vi "Measurement UI.vi"() -> ()   [LabVIEW 2023, in "FPT Intermodulation UI.lvlib"]
uses:
  FPT Intermodulation UI.lvlib
panel:
  in  "Measurement Graph":T1(tab)
  out "Graph Combined":T2(graph)
  out "Graph DUT Gain":T2(graph)
  out "Graph Intermodulation":T2(graph)
  out "Graph TOI":T2(graph)
  out "Graph Fundamental":T2(graph)
  out "TS_Intermodulation Slope (dBm)":dbl[][](array[numeric])
  out "TS_Fundamental Slope (dBm)":dbl[][](array[numeric])
  out "Final Target Pout (dBm)":dbl
  out "All Data":dbl[][](array[numeric])
  out "TS_DUT Gain (dBm)":dbl[][](array[numeric])
  out "TS_TOI (dBm)":dbl[][](array[numeric])
  out "TS_IMD (dBm)":dbl[][](array[numeric])
  out "TS_Fundamental (dBm)":dbl[][](array[numeric])
  out "Typical OIP3 (dBm)":dbl
  out "x-axis label":string
  in  "Power sequencing file path":string
  in  "RFSG name":string="5842_0"
  in  "RFSG attenuation mode":T3(ring)=enum."Constant Attenuation"
  in  "RFSG s2p file path":string
  in  "RFmx name":string="5842_0"
  in  "RFmx attenuation mode":T3(ring)=enum."Constant Attenuation"
  in  "RFmx s2p file path":string
  out "All Graph Reference":refnum<vi>[](array[refnum])
  out "All Plots Data":T4(array[cluster])
  in  "IM_Sweep Mode":enum32{"Power", "Frequency", "Tone Spacing"}(ring) caption="Sweep Mode"
  out "MeasTable_Fix":string[][](table)
  out "MeasTable":string[][](table)
  in  "Tab Control":T5(tab)
  in  "Power sequencing file path_update":path caption="Power Sequencing File Path"
  in  "RFSG name_update":refnum<k15> caption="RFSG Name"
  in  "RFSG attenuation mode_tab":T3(tab)=enum."s2p File" caption="RFSG Attenuation Mode"
  in  "RFSG external attenuation (dB)":dbl caption="External Attenuation" format="%#.3pdB"
  in  "RFSG s2p file path_update":path caption="S2P File Path"
  in  "RFSG s-parameters orientation":enum32{"Port1 Towards DUT", "Port2 Towards DUT"}(ring) caption="Orientation"
  in  "RFmx name_update":refnum<k15> caption="RFmx Name"
  in  "RFmx attenuation mode_tab":T3(tab) caption="RFmx Attenuation Mode"
  in  "RFmx external attenuation (dB)":dbl caption="External Attenuation" format="%#.3pdB"
  in  "RFmx s2p file path_update":path caption="S2P File Path"
  in  "RFmx s-parameters orientation":enum32{"Port1 Towards DUT", "Port2 Towards DUT"}(ring) caption="Orientation"
  in  "RFSG port":string(combo)="port1" caption="RFSG Port"
  in  "RFmx port":string(combo)="port2" caption="RFmx Port"
  in  "RFmx Reference Level (dBm)":dbl=10.0 caption="Reference Level" format="%#.3fdBm"
  in  "RFSG Generation IQ Rate (S/s)":dbl=1250000000.0 caption="Generation IQ Rate" format="%#.3pS/s"
  in  "Start Pin Per Tone (dBm)":dbl=-20.0 caption="Start Pin Per Tone" format="%#.3fdBm"
  in  "Start Center Frequency (Hz)":dbl=8000000000.0 caption="Start Center Frequency" format="%#.3pHz"
  in  "Start Tone Spacing (Hz)":dbl=1000000.0 caption="Start Tone Spacing" format="%#.3pHz"
  in  "Sweep Delay (ms)":u32 format="%#.3pms"
  in  "Sweep Mode_tab":enum32{"Power", "Frequency", "Tone Spacing"}(tab)=enum."Tone Spacing" caption="Sweep Mode"
  in  "Power Sweep End":dbl format="%#.fdBm"
  in  "Power Sweep Step":dbl=1.0 format="%#.fdB"
  in  "Target Pout Per Tone (dBm)":dbl caption="Target Pout Per Tone" format="%#.3fdBm"
  in  "Frequency Sweep End":dbl=12000000000.0 format="%#.pHz"
  in  "Frequency Sweep Step":dbl=100000000.0 format="%#.pHz"
  in  "Tone Spacing Sweep End":dbl=10000000.0 format="%#.pHz"
  in  "Tone Spacing Sweep Step":dbl=1000000.0 format="%#.pHz"
  in  "Mode of operation":T6(ring) caption="Configuration"
  out "Status":string
  # "Intermodulation"
  # "Sweep Options"
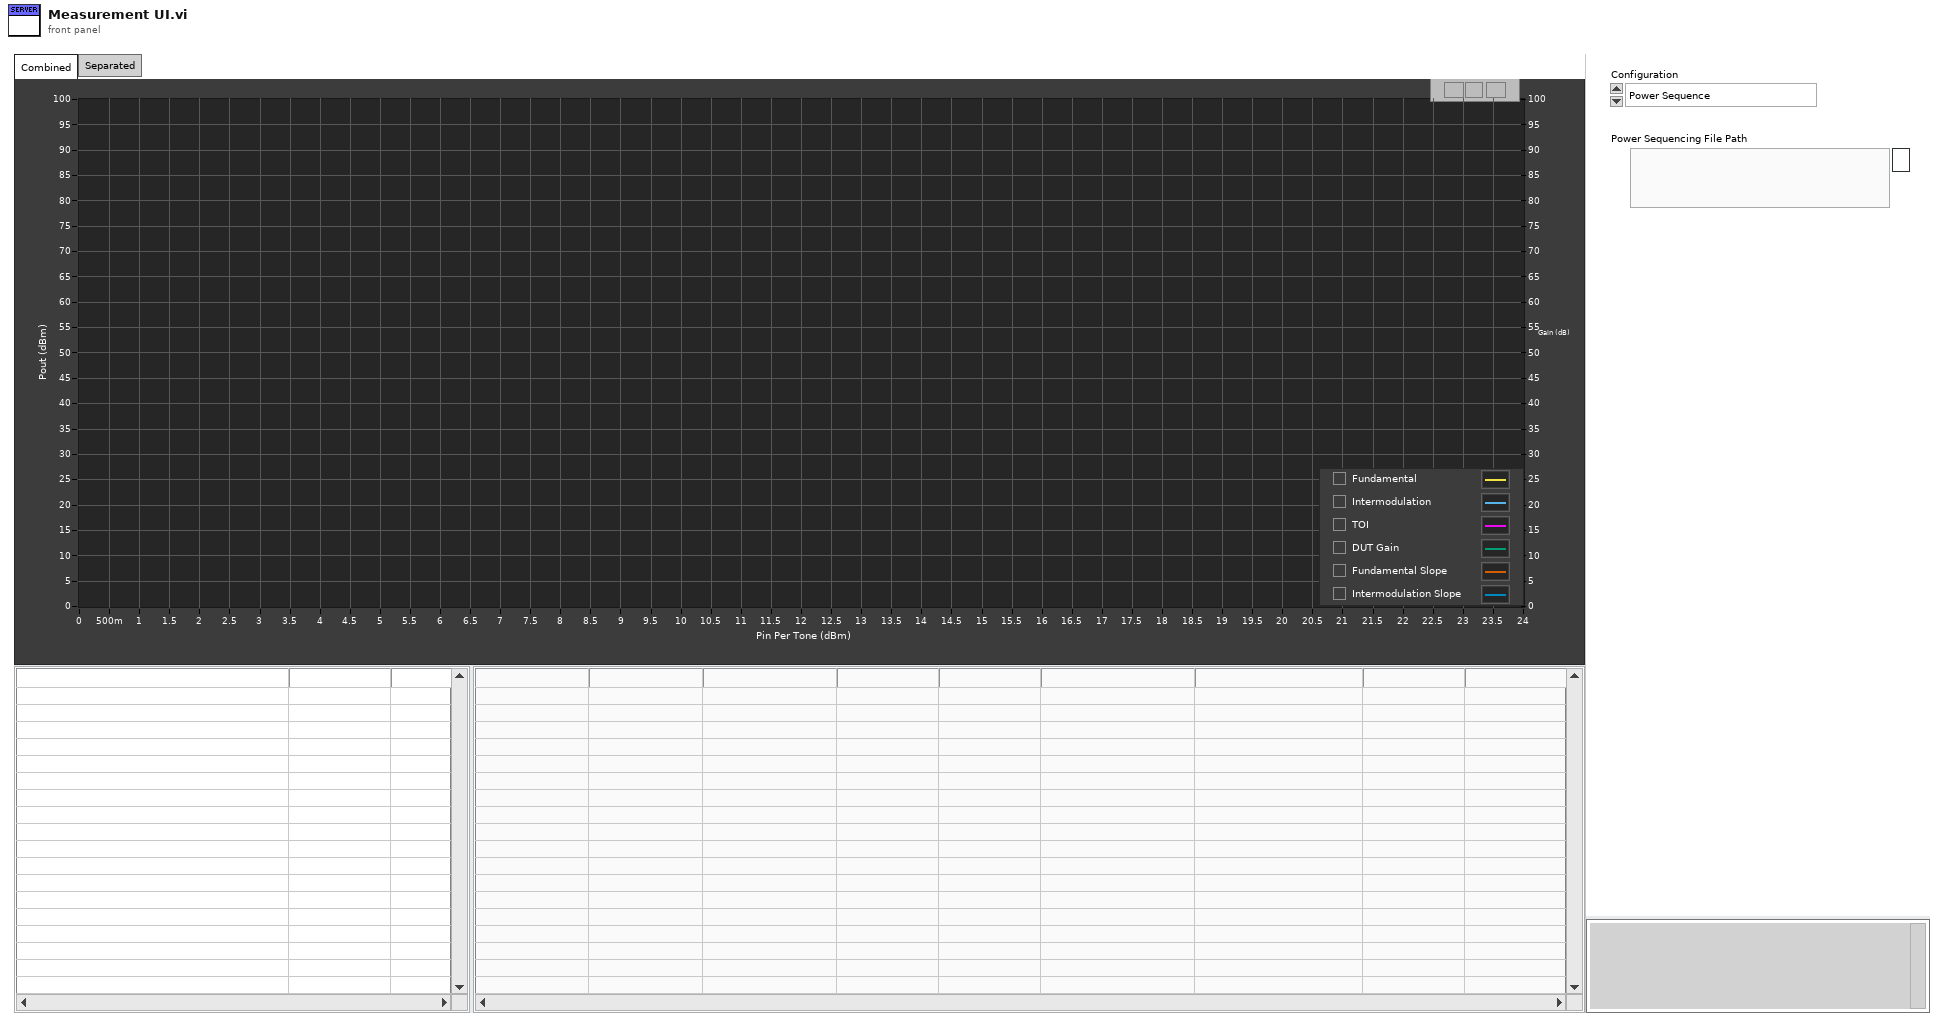
[diagram p1: front panel]
types:
  T1 = enum32{"Combined", "Separated", "Hidden Controls"}
  T2 = cluster{"Load currents":dbl[], "Efficiency":dbl[]}[]
  T3 = enum32{"<None>", "Constant Attenuation", "s2p File"}
  T4 = cluster{"X-axis values":dbl[], "Y-axis values":dbl[]}[]
  T5 = enum32{"Power Sequence", "Correction", "Measurement 1"}
  T6 = enum32{"Power Sequence", "HW + Correction", "Measurement 1"}
  T7 = enum8{"Enabled", "Disabled", "Disabled and Grayed Out"}
  T8 = cluster{"Shift":bool, "Ctrl":bool, "Alt":bool, "Cmd":bool, "Opt":bool}
  T9 = cluster{"TS_Fundamental Slope (dBm)":dbl[], "TS_Fundamental Slope (dBm)":dbl[]}
  T10 = cluster{"TS_Fundamental Slope (dBm)":dbl[], "TS_Intermodulation Slope (dBm)":dbl[]}
  T11 = cluster{"TS_Fundamental Slope (dBm)":dbl[], "TS_Intermodulation Slope (dBm)":dbl[]}[]
  T12 = cluster{"TS_Fundamental (dBm)":dbl[], "TS_Fundamental (dBm)":dbl[]}
  T13 = cluster{"TS_Fundamental (dBm)":dbl[], "TS_IMD (dBm)":dbl[]}
  T14 = cluster{"TS_Fundamental (dBm)":dbl[], "TS_TOI (dBm)":dbl[]}
  T15 = cluster{"TS_Fundamental (dBm)":dbl[], "TS_DUT Gain (dBm)":dbl[]}
  T16 = cluster{"X-axis values":dbl[], "Y-axis values":dbl[]}
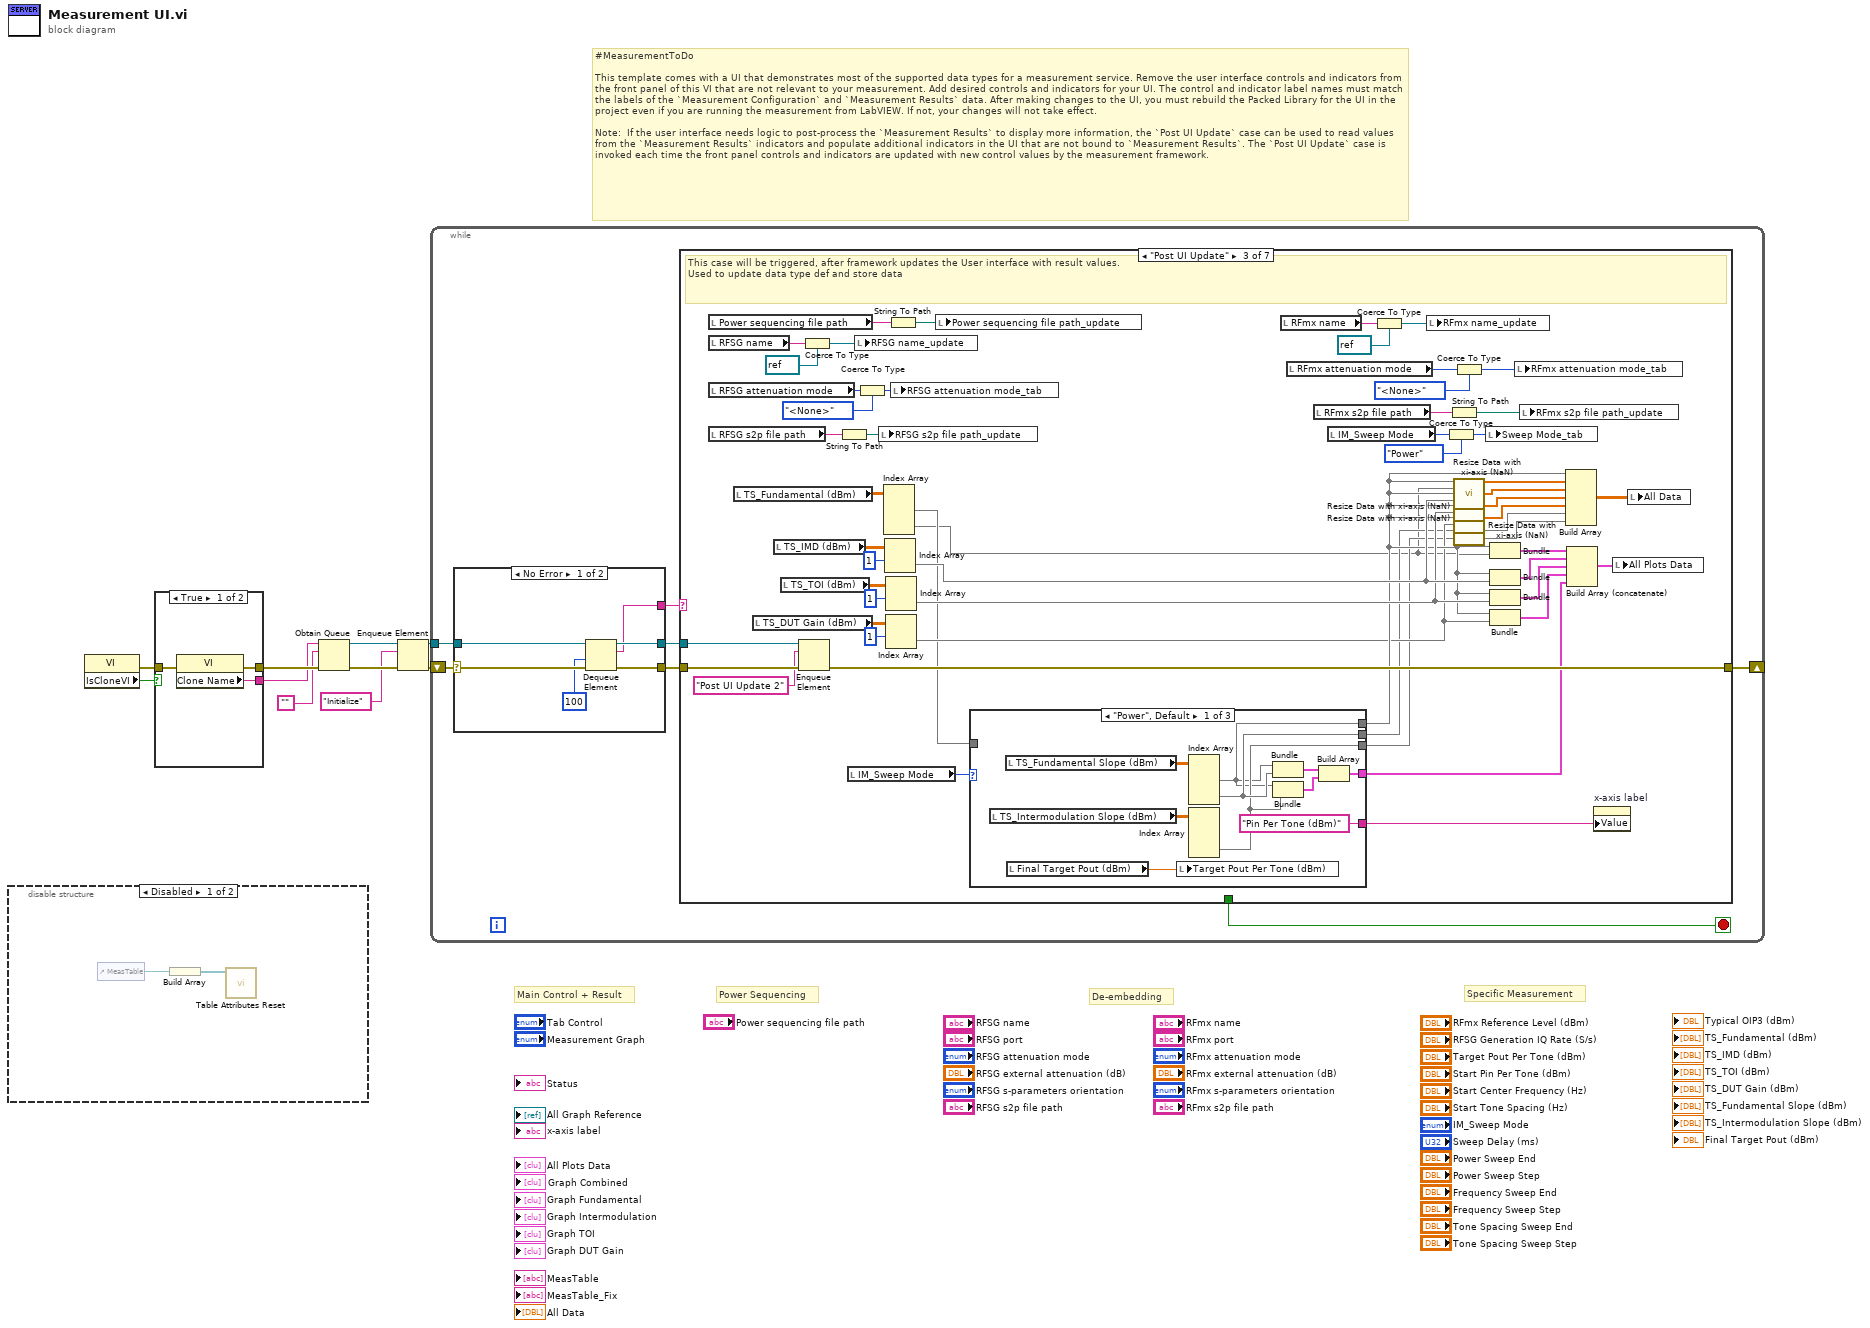
[diagram p0: block diagram]
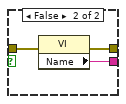
[diagram p3: hidden frame]
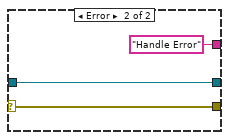
[diagram p4: hidden frame]
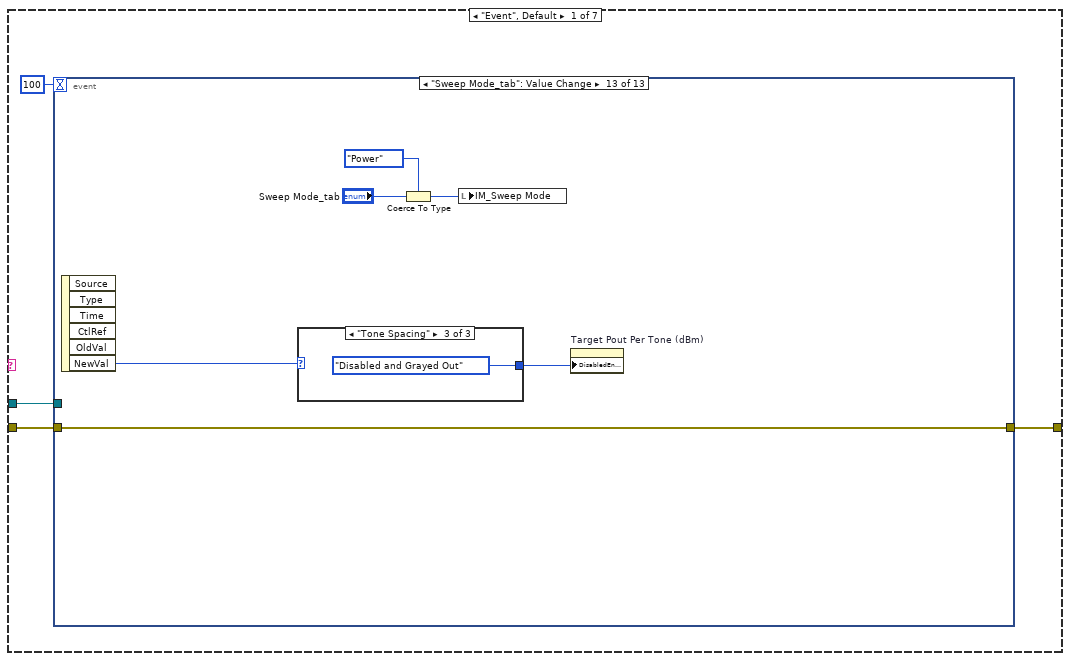
[diagram p5: hidden frame]
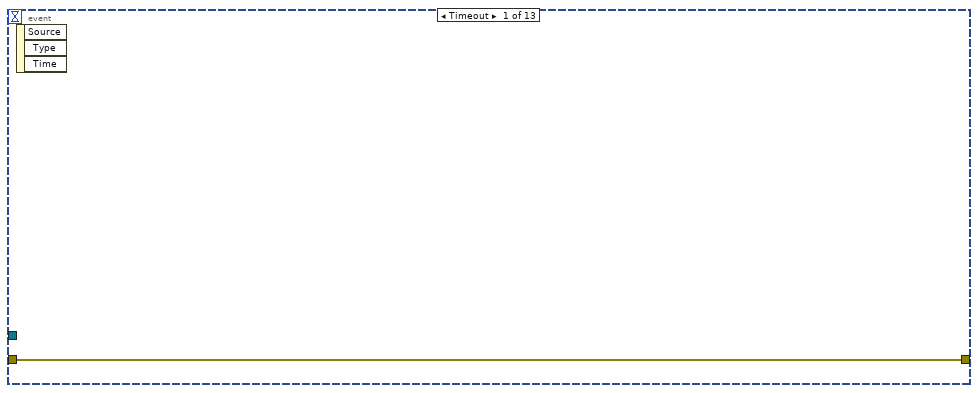
[diagram p6: hidden frame]
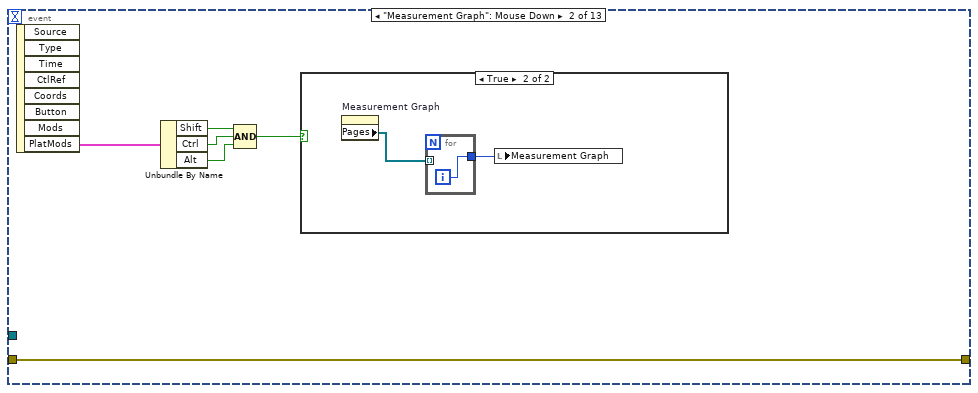
[diagram p7: hidden frame]
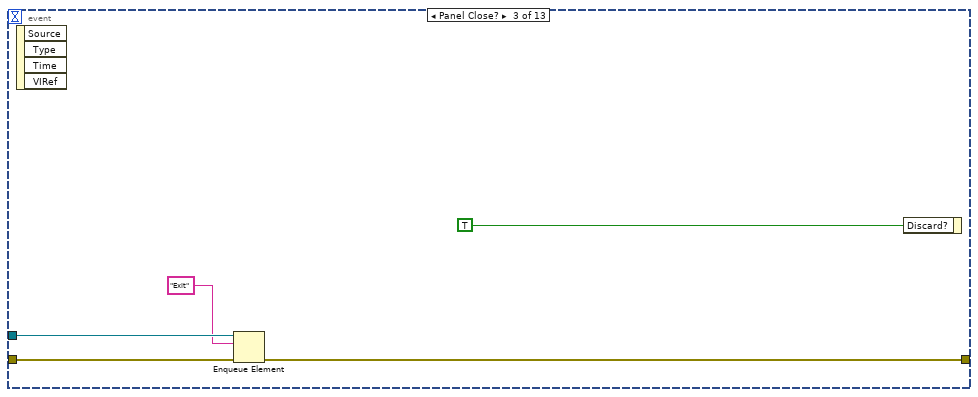
[diagram p9: hidden frame]
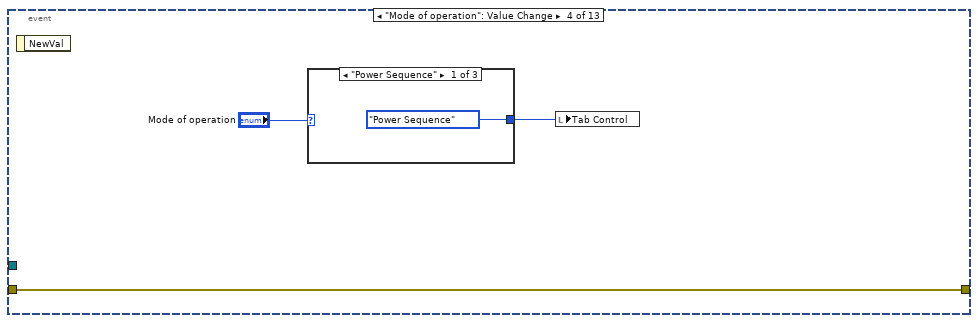
[diagram p10: hidden frame]
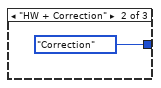
[diagram p11: hidden frame]
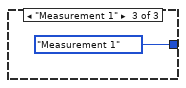
[diagram p12: hidden frame]
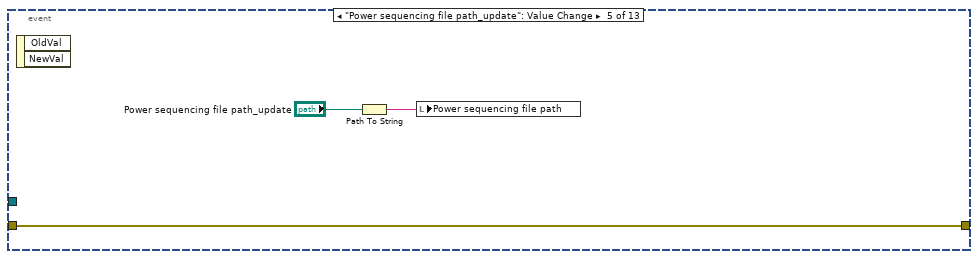
[diagram p13: hidden frame]
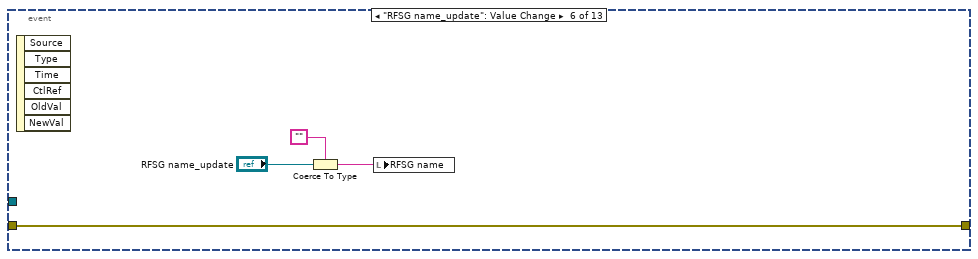
[diagram p14: hidden frame]
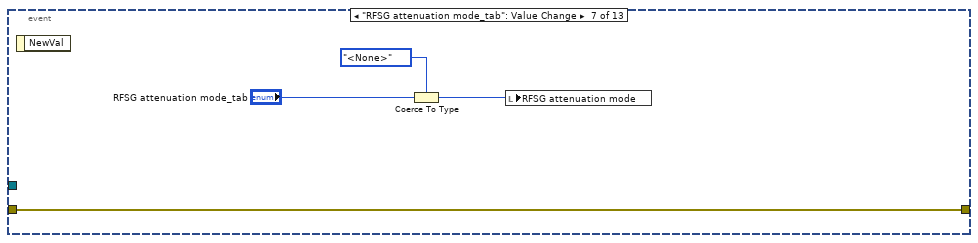
[diagram p15: hidden frame]
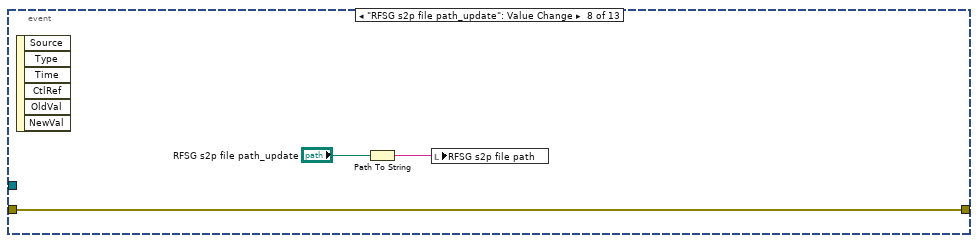
[diagram p16: hidden frame]
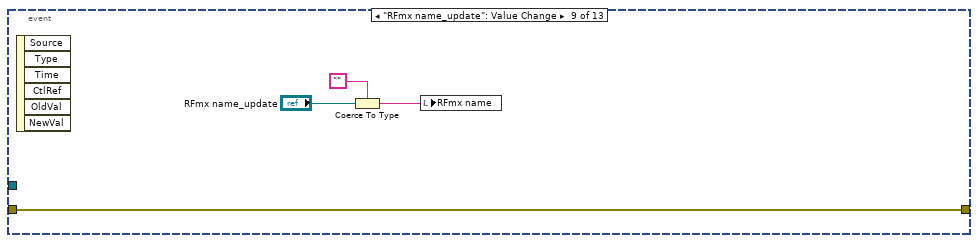
[diagram p17: hidden frame]
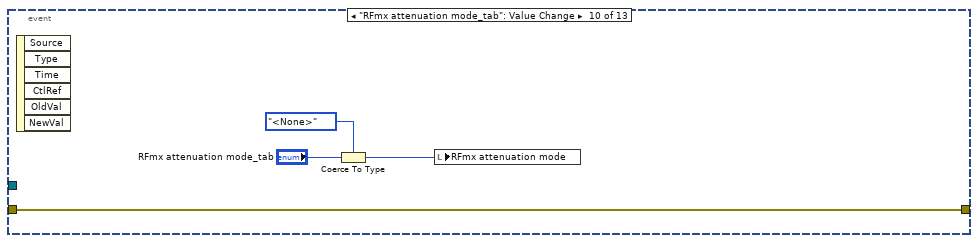
[diagram p18: hidden frame]
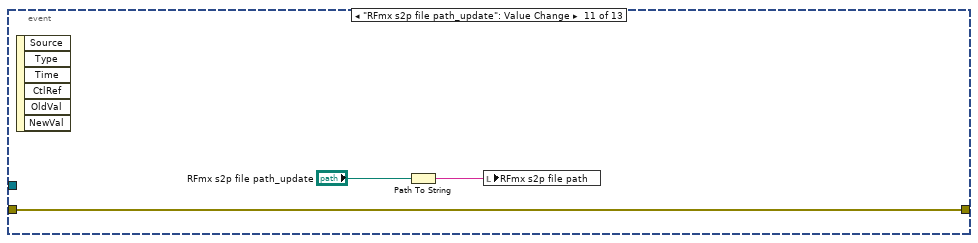
[diagram p19: hidden frame]
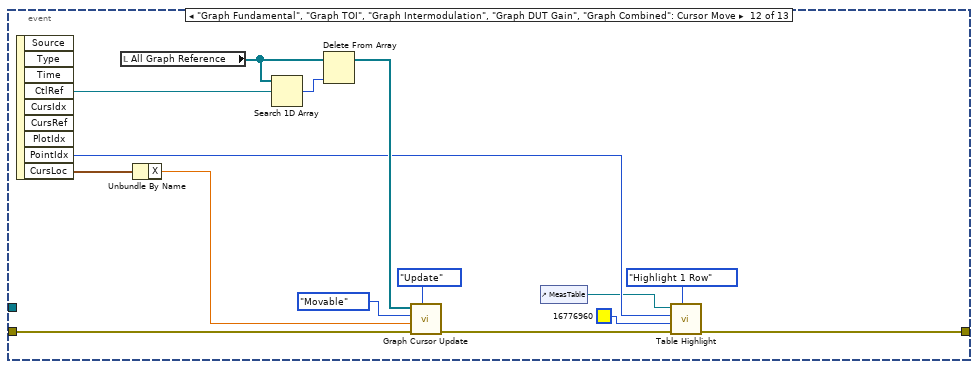
[diagram p20: hidden frame]
diagram:
  # "Specific Measurement"
  # "De-embedding"
  # "Power Sequencing"
  # "Main Control + Result"
  # "#MeasurementToDo  \n\nThis template comes with a UI that demonstrates most of the supported data types for a measurement service. Remove the user interface controls and indicators from the front panel of this VI that are not relevant to your measurement. Add desired controls and indicators for your UI. The control and indicator label names must match the labels of the `Measurement Configuration` and `Measurement Results` data. After making changes to the UI, you must rebuild the Packed Library for the UI in the project even if you are running the measurement from LabVIEW. If not, your changes will not take effect.\n\nNote:  If the user interface needs logic to post-process the `Measurement Results` to display more information, the `Post UI Update` case can be used to read values from the `Measurement Results` indicators and populate additional indicators in the UI that are not bound to `Measurement Results`. The `Post UI Update` case is invoked each time the front panel controls and indicators are updated with new control values by the measurement framework."
  n1 = disable-structure shown="Disabled" {
    frame Disabled {
      n2 = control-ref of="MeasTable"() -> (w12:refnum<vi>)
      n3 = Build Array(w12) -> (w11:refnum<vi>[])
      n4 = call "Table Attributes Reset.vi"("Table Refs"=w11) -> ()  [unwired: 11 in]
    }
    frame Enabled {
    }
  }
  n5 = property class="VI"() -> (error out=w1:errorcluster, "IsCloneVI"=w2:bool)  [unwired: 2 in, 1 out]
  n6 = case shown="True" w2 {
    tunnel: [w15 w18] -> w10
    tunnel: [w14 w17] -> w9
    tunnel: w1 -> [w13 w16]
    frame True {
      n7 = property class="VI"(error in=w13) -> (error out=w15:errorcluster, "Clone Name"=w14:string)  [unwired: 1 in, 1 out]
    }
    frame False {
      n8 = property class="VI"(error in=w16) -> (error out=w18:errorcluster, "Name"=w17:string)  [unwired: 1 in, 1 out]
    }
  }
  n9 = Obtain Queue(name (unnamed)=w9, element data type="", error in (no error)=w10) -> (queue out=w6:refnum<queue>, error out=w8:errorcluster)  [unwired: 2 in, 1 out]
  n10 = Enqueue Element(queue=w6, element="Initialize", error in (no error)=w8) -> (queue out=w5:refnum<queue>, error out=w7:errorcluster)  [unwired: 1 in, 1 out]
  n11 = while {
    shift-right: [w20] -> _
    shift-left: w7 -> [w25]
    tunnel: w5 -> [w23]
    stop <- w19 stop-if-true
    n12 = case shown="No Error" w25 {
      selector: w25 -> [w31 w34]
      tunnel: [w30 w34] -> w24
      tunnel: w23 -> [w29 w33]
      tunnel: [w28 w33] -> w22
      tunnel: [w27 "Handle Error"] -> w21
      frame No Error {
        n13 = Dequeue Element(queue=w29, timeout in ms (-1)=100, error in (no error)=w31) -> (queue out=w28:refnum<queue>, element=w27:string, error out=w30:errorcluster)  [unwired: 1 out]
      }
      frame Error {
      }
    }
    n14 = case shown="\"Post UI Update\"" w21 {
      tunnel: w24 -> [w37 w120 w172 w213 w237 w251 w252]
      tunnel: w22 -> [w35 _ w171 w212 _ w249 _]
      tunnel: [w38 w120 w172 w202 w237 w246 w252] -> w20
      tunnel: [_ _ _ _ _ TRUE _] -> w19
      frame "Event", Default {
        n15 = event shown="[12] \"Sweep Mode_tab\": Value Change" {
          selector: _ -> [_ _ _ _ _ _ _ _ _ _ _ _ _]
          dyn-events: _ -> [_ _ _ _ _ _ _ _ _ _ _ _ _]
          timeout: 100 -> [_ _ _ _ _ _ _ _ _ _ _ _ _]
          tunnel: [w39 w45 w51 w55 w60 w63 w69 w71 w74 w80 w82 w89 w105] -> w38
          tunnel: w37 -> [w39 w45 w52 w55 w60 w63 w69 w71 w74 w80 w82 w99 w105]
          tunnel: w35 -> [_ _ w50 _ _ _ _ _ _ _ _ _ _]
          event Timeout {
            n16 = event-data() -> ()  [unwired: 1 in, 3 out]
          }
          event "Measurement Graph": Mouse Down {
            n17 = event-data() -> ("PlatMods"=w44:T8)  [unwired: 1 in, 7 out]
            n18 = Unbundle By Name(w44) -> ("Shift"=w43:bool, "Ctrl"=w42:bool, "Alt"=w41:bool)
            n19 = Compound Arithmetic op=AND(w43, w42, w41) -> (w40:bool)
            n20 = case shown="True" w40 {
              frame False {
              }
              frame True {
                n21 = property on="Measurement Graph" class="TabCtl (strict)"() -> ("Pages"=w47:refnum<vi>[])  [unwired: 2 in, 2 out]
                n22 = for {
                  tunnel: w47 -> [_] mode=indexing
                  tunnel: [w48] -> w46
                  i -> [w48]
                }
                n23 = local write "Measurement Graph"(w46) -> ()
              }
            }
          }
          event Panel Close? {
            n24 = event-data() -> ()  [unwired: 1 in, 4 out]
            n25 = Enqueue Element(queue=w50, element="Exit", error in (no error)=w52) -> (error out=w51:errorcluster)  [unwired: 1 in, 2 out]
            n26 = event-data("Discard?"=TRUE) -> ()  [unwired: 1 in, 1 out]
          }
          event "Mode of operation": Value Change {
            n27 = event-data() -> ()  [unwired: 1 in, 1 out]
            n28 = case shown="\"Power Sequence\"" "Mode of operation" {
              tunnel: [T5."Power Sequence" ("Tab Control") T5."Correction" ("Tab Control") T5."Measurement 1" ("Tab Control")] -> w54
              frame "Power Sequence" {
              }
              frame "HW + Correction" {
              }
              frame "Measurement 1" {
              }
            }
            n29 = local write "Tab Control"(w54) -> ()
          }
          event "Power sequencing file path_update": Value Change {
            n30 = event-data() -> ()  [unwired: 1 in, 2 out]
            n31 = Path To String(path="Power sequencing file path_update") -> (string=w61:string)
            n32 = local write "Power sequencing file path"(w61) -> ()
          }
          event "RFSG name_update": Value Change {
            n33 = event-data() -> ()  [unwired: 1 in, 6 out]
            n34 = Coerce To Type(0:"RFSG name_update", 1:"") -> (2:w64:string)
            n35 = local write "RFSG name"(w64) -> ()
          }
          event "RFSG attenuation mode_tab": Value Change {
            n36 = event-data() -> ()  [unwired: 1 in, 1 out]
            n37 = Coerce To Type(0:"RFSG attenuation mode_tab", 1:T3."<None>" ("RFSG attenuation mode")) -> (2:w68:T3)
            n38 = local write "RFSG attenuation mode"(w68) -> ()
          }
          event "RFSG s2p file path_update": Value Change {
            n39 = event-data() -> ()  [unwired: 1 in, 6 out]
            n40 = Path To String(path="RFSG s2p file path_update") -> (string=w72:string)
            n41 = local write "RFSG s2p file path"(w72) -> ()
          }
          event "RFmx name_update": Value Change {
            n42 = event-data() -> ()  [unwired: 1 in, 6 out]
            n43 = Coerce To Type(0:"RFmx name_update", 1:"") -> (2:w76:string)
            n44 = local write "RFmx name"(w76) -> ()
          }
          event "RFmx attenuation mode_tab": Value Change {
            n45 = event-data() -> ()  [unwired: 1 in, 6 out]
            n46 = Coerce To Type(0:"RFmx attenuation mode_tab", 1:T3."<None>" ("RFmx attenuation mode")) -> (2:w79:T3)
            n47 = local write "RFmx attenuation mode"(w79) -> ()
          }
          event "RFmx s2p file path_update": Value Change {
            n48 = event-data() -> ()  [unwired: 1 in, 6 out]
            n49 = Path To String(path="RFmx s2p file path_update") -> (string=w83:string)
            n50 = local write "RFmx s2p file path"(w83) -> ()
          }
          event "Graph Fundamental", "Graph TOI", "Graph Intermodulation", "Graph DUT Gain", "Graph Combined": Cursor Move {
            n51 = event-data() -> ("CtlRef"=w97:refnum<vi>, "PointIdx"=w87:i32, "CursLoc"=w98:cluster{"X":dbl, "Y":dbl})  [unwired: 1 in, 6 out]
            n52 = local read "All Graph Reference"() -> (w96:refnum<vi>[])
            n53 = Unbundle By Name(w98) -> ("X"=w92:dbl)
            n54 = Search 1D Array(1D array=w96, element=w97) -> (index of element=w95:i32)  [unwired: 1 in]
            n55 = Delete From Array(array=w96, index=w95) -> (array with subset deleted=w94:refnum<vi>[])  [unwired: 1 in, 1 out]
            n56 = call "Graph Cursor Update.vi"("Action"=enum16{"Reset", "Update"}."Update", "error in"=w99, "New X position"=w92, "Cursor Type"=enum16{"Movable", "Fixed", "All"}."Movable", "Graph Refs in"=w94) -> ("error out"=w90:errorcluster)  [unwired: 5 in, 1 out]
            n57 = control-ref of="MeasTable"() -> (w86:refnum<vi>)
            n58 = call "Table Highlight.vi"("Action"=enum16{"Reset", "Highlight 1 Row"}."Highlight 1 Row", "error in"=w90, "Color Box"=u32 16776960, "Row"=w87, "Table Ref in"=w86) -> ("error out"=w89:errorcluster)  [unwired: 5 in, 1 out]
          }
          event "Sweep Mode_tab": Value Change {
            n59 = event-data() -> ("NewVal"=w100:enum32{"Power", "Frequency", "Tone Spacing"})  [unwired: 1 in, 5 out]
            n60 = case shown="\"Tone Spacing\"" w100 {
              tunnel: [T7."Disabled and Grayed Out" ("Disabled") T7."Enabled" ("Disabled") T7."Disabled and Grayed Out" ("Disabled")] -> w101
              frame "Frequency" {
              }
              frame "Power" {
              }
              frame "Tone Spacing" {
              }
            }
            n61 = Coerce To Type(0:"Sweep Mode_tab", 1:enum32{"Power", "Frequency", "Tone Spacing"}."Power" ("IM_Sweep Mode")) -> (2:w102:enum32{"Power", "Frequency", "Tone Spacing"})
            n62 = local write "IM_Sweep Mode"(w102) -> ()
            n63 = property on="Target Pout Per Tone (dBm)" class="DigNum (strict)"("DisabledEnum"=w101) -> ()  [unwired: 2 in, 2 out]
          }
        }
      }
      frame "Initialize" {
        w115 = 0
        n64 = local write "Tab Control"(w115) -> ()
        n65 = local write "Mode of operation"(w115) -> ()
        n66 = control-ref of="Graph Combined"() -> (w114:refnum<vi>)
        n67 = control-ref of="Graph Fundamental"() -> (w119:refnum<vi>)
        n68 = control-ref of="Graph Intermodulation"() -> (w117:refnum<vi>)
        n69 = control-ref of="Graph TOI"() -> (w116:refnum<vi>)
        n70 = control-ref of="Graph DUT Gain"() -> (w118:refnum<vi>)
        n71 = Build Array(w114, w119, w117, w116, w118) -> (w113:refnum<vi>[])
        n72 = property on="All Graph Reference" class="Arr (strict)"("Value"=w113) -> ()  [unwired: 2 in, 2 out]
        n73 = call "Graph Set Cursor Mode.vi"("Cursor Mode"=enum32{"Free-Drag", "Single-Plot", "Multi-Plot"}."Multi-Plot", "Graph Refs in"=w113) -> ("Graph Refs out"=w111:refnum<vi>[])  [unwired: 8 in, 1 out]
        n74 = call "Graph Cursor Update.vi"("Action"=enum16{"Reset", "Update"}."Reset", "Cursor Type"=enum16{"Movable", "Fixed", "All"}."All", "Graph Refs in"=w111) -> ()  [unwired: 7 in, 2 out]
      }
      frame "Post UI Update" {
        # "This case will be triggered, after framework updates the User interface with result values.\nUsed to update data type def and store data"
        n75 = local read "Power sequencing file path"() -> (w168:string)
        n76 = local read "RFSG name"() -> (w166:string)
        n77 = local read "RFSG attenuation mode"() -> (w167:T3)
        n78 = local read "RFSG s2p file path"() -> (w162:string)
        n79 = local read "TS_Fundamental (dBm)"() -> (w122:dbl[][])
        n80 = local read "TS_DUT Gain (dBm)"() -> (w149:dbl[][])
        n81 = local read "TS_IMD (dBm)"() -> (w151:dbl[][])
        n82 = local read "TS_TOI (dBm)"() -> (w150:dbl[][])
        n83 = Enqueue Element(queue=w171, element="Post UI Update 2") -> ()  [unwired: 2 in, 3 out]
        n84 = Coerce To Type(0:w166, 1:refnum<k15> refnum ("RFSG name_update")) -> (2:w164:refnum<k15>)
        n85 = String To Path(string=w162) -> (path=w163:path)
        n86 = local read "IM_Sweep Mode"() -> (w123:enum32{"Power", "Frequency", "Tone Spacing"})
        n87 = local write "RFSG name_update"(w164) -> ()
        n88 = Coerce To Type(0:w167, 1:T3."<None>" ("RFSG attenuation mode_tab")) -> (2:w155:T3)
        n89 = local write "RFSG s2p file path_update"(w163) -> ()
        n90 = Index Array(array=w122) -> (element #1=w130:dbl[], element #2=w121:dbl[])  [unwired: 4 in]
        n91 = Index Array(array=w151, index (row)=1) -> (element=w138:dbl[])  [unwired: 1 in]
        n92 = Index Array(array=w150, index (row)=1) -> (element=w136:dbl[])  [unwired: 1 in]
        n93 = Index Array(array=w149, index (row)=1) -> (element=w133:dbl[])  [unwired: 1 in]
        n94 = String To Path(string=w168) -> (path=w169:path)
        n95 = local write "RFSG attenuation mode_tab"(w155) -> ()
        n96 = local write "Power sequencing file path_update"(w169) -> ()
        n97 = case shown="\"Power\", Default" w123 {
          tunnel: [w180 _ _] -> w132
          tunnel: [w177 _ _] -> w141
          tunnel: w130 -> [_ w183 w185]
          tunnel: [w179 _ _] -> w131
          tunnel: ["Pin Per Tone (dBm)" "Frequency (GHz)" "Tone Spacing (MHz)"] -> w148
          tunnel: [w174 w183 w185] -> w134
          frame "Power", Default {
            n98 = local read "TS_Intermodulation Slope (dBm)"() -> (w181:dbl[][])
            n99 = local read "TS_Fundamental Slope (dBm)"() -> (w182:dbl[][])
            n100 = local read "Final Target Pout (dBm)"() -> (w173:dbl)
            n101 = local write "Target Pout Per Tone (dBm)"(w173) -> ()
            n102 = Index Array(array=w182) -> (element #1=w174:dbl[], element #2=w180:dbl[])  [unwired: 4 in]
            n103 = Index Array(array=w181) -> (element #2=w179:dbl[])  [unwired: 4 in, 1 out]
            n104 = Bundle("TS_Fundamental Slope (dBm)"=w174, "TS_Fundamental Slope (dBm)"=w180) -> (w178:T9)  [unwired: 1 in]
            n105 = Bundle("TS_Fundamental Slope (dBm)"=w174, "TS_Intermodulation Slope (dBm)"=w179) -> (w176:T10)  [unwired: 1 in]
            n106 = Build Array(w178, w176) -> (w177:T11)
          }
          frame "Frequency" {
          }
          frame "Tone Spacing" {
          }
        }
        n107 = local read "RFmx name"() -> (w157:string)
        n108 = local read "RFmx attenuation mode"() -> (w156:T3)
        n109 = local read "RFmx s2p file path"() -> (w161:string)
        n110 = local read "IM_Sweep Mode"() -> (w129:enum32{"Power", "Frequency", "Tone Spacing"})
        n111 = Coerce To Type(0:w157, 1:refnum<k15> refnum ("RFSG name_update")) -> (2:w159:refnum<k15>)
        n112 = local write "RFmx name_update"(w159) -> ()
        n113 = Coerce To Type(0:w129, 1:enum32{"Power", "Frequency", "Tone Spacing"}."Power" ("Sweep Mode_tab")) -> (2:w127:enum32{"Power", "Frequency", "Tone Spacing"})
        n114 = String To Path(string=w161) -> (path=w160:path)
        n115 = Coerce To Type(0:w156, 1:T3."<None>" ("RFmx attenuation mode_tab")) -> (2:w153:T3)
        n116 = call "Resize Data with xi-axis (NaN).vi"("x-axis"=w134, "Measure data"=w121) -> ("Updated Data"=w140:dbl[])  [unwired: 13 in]
        n117 = call "Resize Data with xi-axis (NaN).vi"("x-axis"=w134, "Measure data"=w138) -> ("Updated Data"=w139:dbl[])  [unwired: 13 in]
        n118 = call "Resize Data with xi-axis (NaN).vi"("x-axis"=w134, "Measure data"=w136) -> ("Updated Data"=w137:dbl[])  [unwired: 13 in]
        n119 = call "Resize Data with xi-axis (NaN).vi"("x-axis"=w134, "Measure data"=w133) -> ("Updated Data"=w135:dbl[])  [unwired: 13 in]
        n120 = local write "Sweep Mode_tab"(w127) -> ()
        n121 = Bundle("TS_Fundamental (dBm)"=w134, "TS_Fundamental (dBm)"=w121) -> (w145:T12)  [unwired: 1 in]
        n122 = Bundle("TS_Fundamental (dBm)"=w134, "TS_IMD (dBm)"=w138) -> (w144:T13)  [unwired: 1 in]
        n123 = Bundle("TS_Fundamental (dBm)"=w134, "TS_TOI (dBm)"=w136) -> (w143:T14)  [unwired: 1 in]
        n124 = Bundle("TS_Fundamental (dBm)"=w134, "TS_DUT Gain (dBm)"=w133) -> (w142:T15)  [unwired: 1 in]
        n125 = local write "RFmx attenuation mode_tab"(w153) -> ()
        n126 = local write "RFmx s2p file path_update"(w160) -> ()
        n127 = Build Array(w134, w140, w139, w137, w135, w132, w131) -> (w147:dbl[][])
        n128 = Build Array (concatenate)(w145, w144, w143, w142, w141) -> (w146:T11)
        n129 = property on="x-axis label" class="Str"("Value"=w148) -> ()  [unwired: 2 in, 2 out]
        n130 = local write "All Plots Data"(w146) -> ()
        n131 = local write "All Data"(w147) -> ()
      }
      frame "Post UI Update 2" {
        # "#ToBeImprove\n- highlight or bold the row with expected Pout\n- hide the cursor when not using power sweep"
        # "update Target Pout Per Tone"
        # "Run after Post UI Update. Can be duplicate is need more processing.\nUpdate all data to graph"
        n132 = Enqueue Element(queue=w212, element="Post UI Update 3", error in (no error)=w213) -> (error out=w190:errorcluster)  [unwired: 1 in, 2 out]
        n133 = local read "All Graph Reference"() -> (w188:refnum<vi>[])
        n134 = local read "All Plots Data"() -> (w198:T4)
        n135 = local read "x-axis label"() -> (w187:string)
        n136 = control-ref of="Graph Combined"() -> (w201:refnum<vi>)
        n137 = Build Array(w201) -> (w200:refnum<vi>[])
        n138 = for {
          tunnel: w188 -> [w216] mode=indexing
          shift-right: [w217] -> w189
          shift-left: w190 -> [w218]
          tunnel: w187 -> [w215]
          n139 = property class="XYGraph (strict)"(reference=w216, error in=w218, "XScale.NameLbl.Text"=w215) -> (error out=w217:errorcluster)  [unwired: 1 out]
        }
        n140 = call "Graph Update.vi"("Graph Type"=enum16{"Combined", "Multiple"}."Combined", "Graph Plots"=w198, "Graph Reference in"=w200) -> ()  [unwired: 8 in, 1 out]
        n141 = local read "Target Pout Per Tone (dBm)"() -> (w210:dbl)
        n142 = local read "All Plots Data"() -> (w209:T4)
        n143 = local read "x-axis label"() -> (w211:string)
        n144 = control-ref of="Graph Fundamental"() -> (w197:refnum<vi>)
        n145 = control-ref of="Graph Intermodulation"() -> (w196:refnum<vi>)
        n146 = control-ref of="Graph TOI"() -> (w195:refnum<vi>)
        n147 = control-ref of="Graph DUT Gain"() -> (w194:refnum<vi>)
        n148 = Index Array(array=w209) -> (element=w208:T16)  [unwired: 1 in]
        n149 = local read "All Plots Data"() -> (w191:T4)
        n150 = call "Get Pin at Target Pout.vi"("error in"=w189, "x-axis name"=w211, "IM_Target Pout Per Tone (dBm)"=w210, "Graph Data"=w208) -> ("error out"=w207:errorcluster, "Pin @ Target Pout"=w203:dbl)  [unwired: 6 in]
        n151 = Build Array(w197, w196, w195, w194) -> (w193:refnum<vi>[])
        n152 = local read "All Graph Reference"() -> (w205:refnum<vi>[])
        n153 = call "Graph Update.vi"("Graph Type"=enum16{"Combined", "Multiple"}."Multiple", "Graph Plots"=w191, "Graph Reference in"=w193) -> ()  [unwired: 8 in, 1 out]
        n154 = call "Graph Cursor Update.vi"("Action"=enum16{"Reset", "Update"}."Update", "error in"=w207, "New X position"=w203, "Cursor Type"=enum16{"Movable", "Fixed", "All"}."Fixed", "Graph Refs in"=w205) -> ("error out"=w202:errorcluster)  [unwired: 5 in, 1 out]
      }
      frame "Post UI Update 3" {
        # "Run after Post UI Update. Can be duplicate is need more processing.\nUpdate data into table"
        n155 = local read "x-axis label"() -> (w233:string)
        n156 = Equal?(x=w233, y="Pin Per Tone (dBm)") -> (x = y?=w223:bool)
        n157 = case shown="True" w223 {
          tunnel: [w239 string[] ["Fundamental Slope (dBm)", "Intermodulation Slope (dBm)"]] -> w222
          tunnel: [2 ("length") 0 ("length")] -> w219
          frame False {
            n158 = Build Array("") -> (w239:string[])
          }
          frame True {
          }
        }
        n159 = case shown="False" w223 {
          tunnel: [string[] ["Output Third-Order Intercept (OIP3)"] string[] ["Typical Output Third-Order Intercept (OIP3)"]] -> w232
          frame True {
          }
          frame False {
          }
        }
        n160 = local read "x-axis label"() -> (w226:string)
        n161 = local read "Typical OIP3 (dBm)"() -> (w231:dbl)
        n162 = Build Array (concatenate)(w226, string[] ["Fundamental (dBm)", "Intermodulation (dBm)", "TOI (dBm)", "DUT Gain (dBm)"], w222) -> (w224:string[])
        n163 = local read "All Data"() -> (w221:dbl[][])
        n164 = Build Array(w231) -> (w230:dbl[])
        n165 = control-ref of="MeasTable_Fix"() -> (w235:refnum<vi>)
        n166 = control-ref of="MeasTable"() -> (w236:refnum<vi>)
        n167 = Build Array(w230) -> (w229:dbl[][])
        n168 = Delete From Array(array=w221, length=w219) -> (array with subset deleted=w220:dbl[][])  [unwired: 2 in, 1 out]
        n169 = call "Table Set Header Name and Data (DBL).vi"("format string"="%#.3p" ("Results Num Format"), "Data"=w229, "Header"=w232, "Table Ref"=w235) -> ()  [unwired: 8 in]
        n170 = call "Table Set Header Name and Data (DBL).vi"("format string"="%#.3p" ("Results Num Format"), "Data"=w220, "Header"=w224, "Table Ref"=w236) -> ()  [unwired: 8 in]
      }
      frame "Exit" {
        # "This case is triggered to close the User Interface from framework"
        n171 = Flush Queue(queue=w249, error in (no error)=w251) -> (queue out=w248:refnum<queue>, error out=w247:errorcluster)  [unwired: 1 out]
        n172 = Release Queue(queue=w248, force destroy? (F)=TRUE, error in (no error)=w247) -> (error out=w246:errorcluster)  [unwired: 2 out]
      }
      frame "Handle Error" {
      }
    }
  }
